vi "to_json.vi"(8 "error in":errorcluster, 11 "trueFrameRate in":refnum<class "trueFrameRate.lvclass">) -> (0 "error out":errorcluster, 2 "json":string, 3 "trueFrameRate out":refnum<class "trueFrameRate.lvclass">, 4 "Not Default":bool)   [LabVIEW 2020, in "nominal types.lvlib" / "timestampManifest.lvlib" / "trueFrameRate.lvclass"]
uses:
  trueFrameRate.lvclass
  trueFrameRate.lvclass/trueFrameRate.ctl
  3737468a-64db-419b-9e6c-8f4439dbebd7.vi
  <vilib>/JDP Science/JSONtext/Variant to JSON Text.vi
  <vilib>/JDP Science/JSONtext/LVClass Serializer/JSONtext LVClass Serializer.lvclass
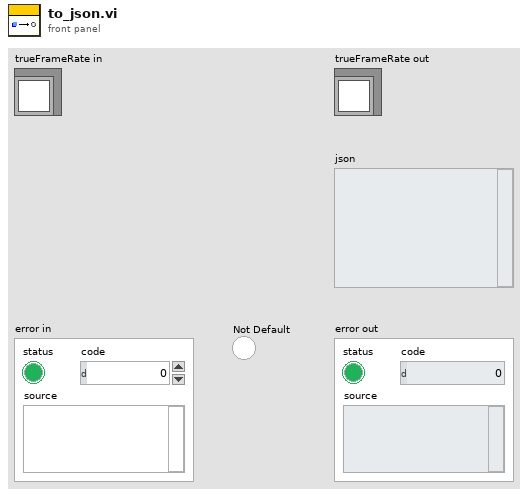
[diagram p1: front panel]
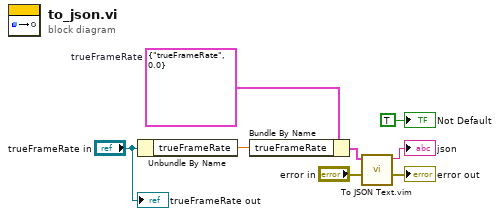
[diagram p0: block diagram]
diagram:
  w7 = cluster{"type":string, "trueFrameRate":dbl} {"type"="trueFrameRate", "trueFrameRate"=0.0}  # trueFrameRate
  n1 = Unbundle By Name("trueFrameRate in") -> ("trueFrameRate"=w6:dbl)
  n2 = Bundle By Name(cluster=w7, "trueFrameRate"=w6) -> (w5:cluster{"type":string, "trueFrameRate":dbl})
  n3 = call "To JSON Text.vim"("error in (no error)"="error in", "Anything"=w5) -> ("error out"=→"error out":errorcluster, "<JSON>"=→"json":string)  [unwired: 8 in]
  "trueFrameRate out" <- "trueFrameRate in"
  "Not Default" <- TRUE ("Not Default")
